vi "Hang Controller.vi"(8 "error in":errorcluster) -> ()   [LabVIEW 2019]
doc: "This VI executes continuously carrying out the current operation and responding to updates or new operations. It will often contain the timing or control code that is difficult to place directly in TeleOp. This VI generally opens all sensors and motors and isolates the rest of the robot code from knowing how the operations are carried out."
uses:
  <vilib>/Rock Robotics/WPI/Framework/Completion Status.ctl
  Hang Setpoints.ctl
  Hang Operations.ctl
  <vilib>/Rock Robotics/SystemInterfaces/DIO/FPGA_DIOPWMChannel.ctl
  <vilib>/Rock Robotics/WPI/ThirdParty/Phoenix-LabVIEW/Motor Controller/Controls/CTRE_Phoenix_MotorControl_NeutralMode.ctl
  <vilib>/Rock Robotics/WPI/ThirdParty/Phoenix-LabVIEW/Motor Controller/Controls/CTRE_Phoenix_MotorControl_TalonFXMotorControllerConfigurables.ctl
  <vilib>/Rock Robotics/WPI/ThirdParty/Phoenix-LabVIEW/Motor Controller/Controls/CTRE_Phoenix_MotorControl_BaseConfigurables.ctl
  <vilib>/Rock Robotics/WPI/ThirdParty/Phoenix-LabVIEW/Motor Controller/Controls/CTRE_Phoenix_MotorControl_VelocityMeasurementPeriod.ctl
  <vilib>/Rock Robotics/WPI/ThirdParty/Phoenix-LabVIEW/Motor Controller/Controls/CTRE_Phoenix_MotorControl_SlotStructure.ctl
  <vilib>/Rock Robotics/WPI/ThirdParty/Phoenix-LabVIEW/Motor Controller/Controls/CTRE_Phoenix_MotorControl_FilterStruct.ctl
  <vilib>/Rock Robotics/WPI/ThirdParty/Phoenix-LabVIEW/Motor Controller/Controls/CTRE_Phoenix_MotorControl_RemoteSourceType.ctl
  <vilib>/Rock Robotics/WPI/ThirdParty/Phoenix-LabVIEW/Controls/CTRE_Phoenix_CustomParamConfiguration.ctl
  <vilib>/Rock Robotics/WPI/ThirdParty/Phoenix-LabVIEW/Motor Controller/Controls/CTRE_Phoenix_MotorControl_FeedbackDevice_TalonFX.ctl
  <vilib>/Rock Robotics/WPI/ThirdParty/Phoenix-LabVIEW/Motor Controller/Controls/CTRE_Phoenix_MotorControl_LimitSwitchNormal.ctl
  <vilib>/Rock Robotics/WPI/ThirdParty/Phoenix-LabVIEW/Motor Controller/Controls/CTRE_Phoenix_MotorControl_LimitSwitchSource_Local.ctl
  <vilib>/Rock Robotics/WPI/ThirdParty/Phoenix-LabVIEW/Motor Controller/Controls/CTRE_Phoenix_MotorControl_SupplyCurrentLimitConfiguration.ctl
  <vilib>/Rock Robotics/WPI/ThirdParty/Phoenix-LabVIEW/Motor Controller/Controls/CTRE_Phoenix_MotorControl_StatorCurrentLimitConfiguration.ctl
  <vilib>/Rock Robotics/WPI/ThirdParty/Phoenix-LabVIEW/Motor Controller/Controls/CTRE_Phoenix_MotorControl_MotorCommutation_TalonFX.ctl
  <vilib>/Rock Robotics/WPI/ThirdParty/Phoenix-LabVIEW/CANCoder/Controls/CTRE_Phoenix_CANcoder_AbsoluteSensorRange.ctl
  <vilib>/Rock Robotics/WPI/ThirdParty/Phoenix-LabVIEW/CANCoder/Controls/CTRE_Phoenix_CANcoder_SensorInitializationStrategy.ctl
  <vilib>/Rock Robotics/WPI/ThirdParty/Phoenix-LabVIEW/Motor Controller/Controls/CTRE_Phoenix_MotorControl_ControlMode.ctl
  <vilib>/Rock Robotics/WPI/ThirdParty/Phoenix-LabVIEW/Motor Controller/Get/CTRE_Phoenix_MotorController_GetSelectedSensorData.vi
  <vilib>/Rock Robotics/WPI/ThirdParty/Phoenix-LabVIEW/Motor Controller/Get/CTRE_Phoenix_MotorController_GetSupplyAndStatorCurrent_Enhanced.vi
  Framework/Robot Global Data.vi
  <vilib>/Rock Robotics/Network Tables/NT Write Boolean.vi
panel:
  in  "Interactive Values":T1
  out "Current\nCmd":string
  in  "Buttons":cluster{"Execute Cmd":bool, "Abort Cmd":bool}
  out "Command Timing":cluster{"Start Time (ms)":u32, "Iterations":i32}
  out "Status":T3
  # "Tip: It may be helpful to observe inputs and sensor values.\nYou may also want to display tuning or debugging controls."
  # "Up"
  # "Down"
  # "Interactive Command: You may fill in the settings for a command\nand schedule it with the Execute button. You can observe and abort\nany command while fine tuning the code for the controller."
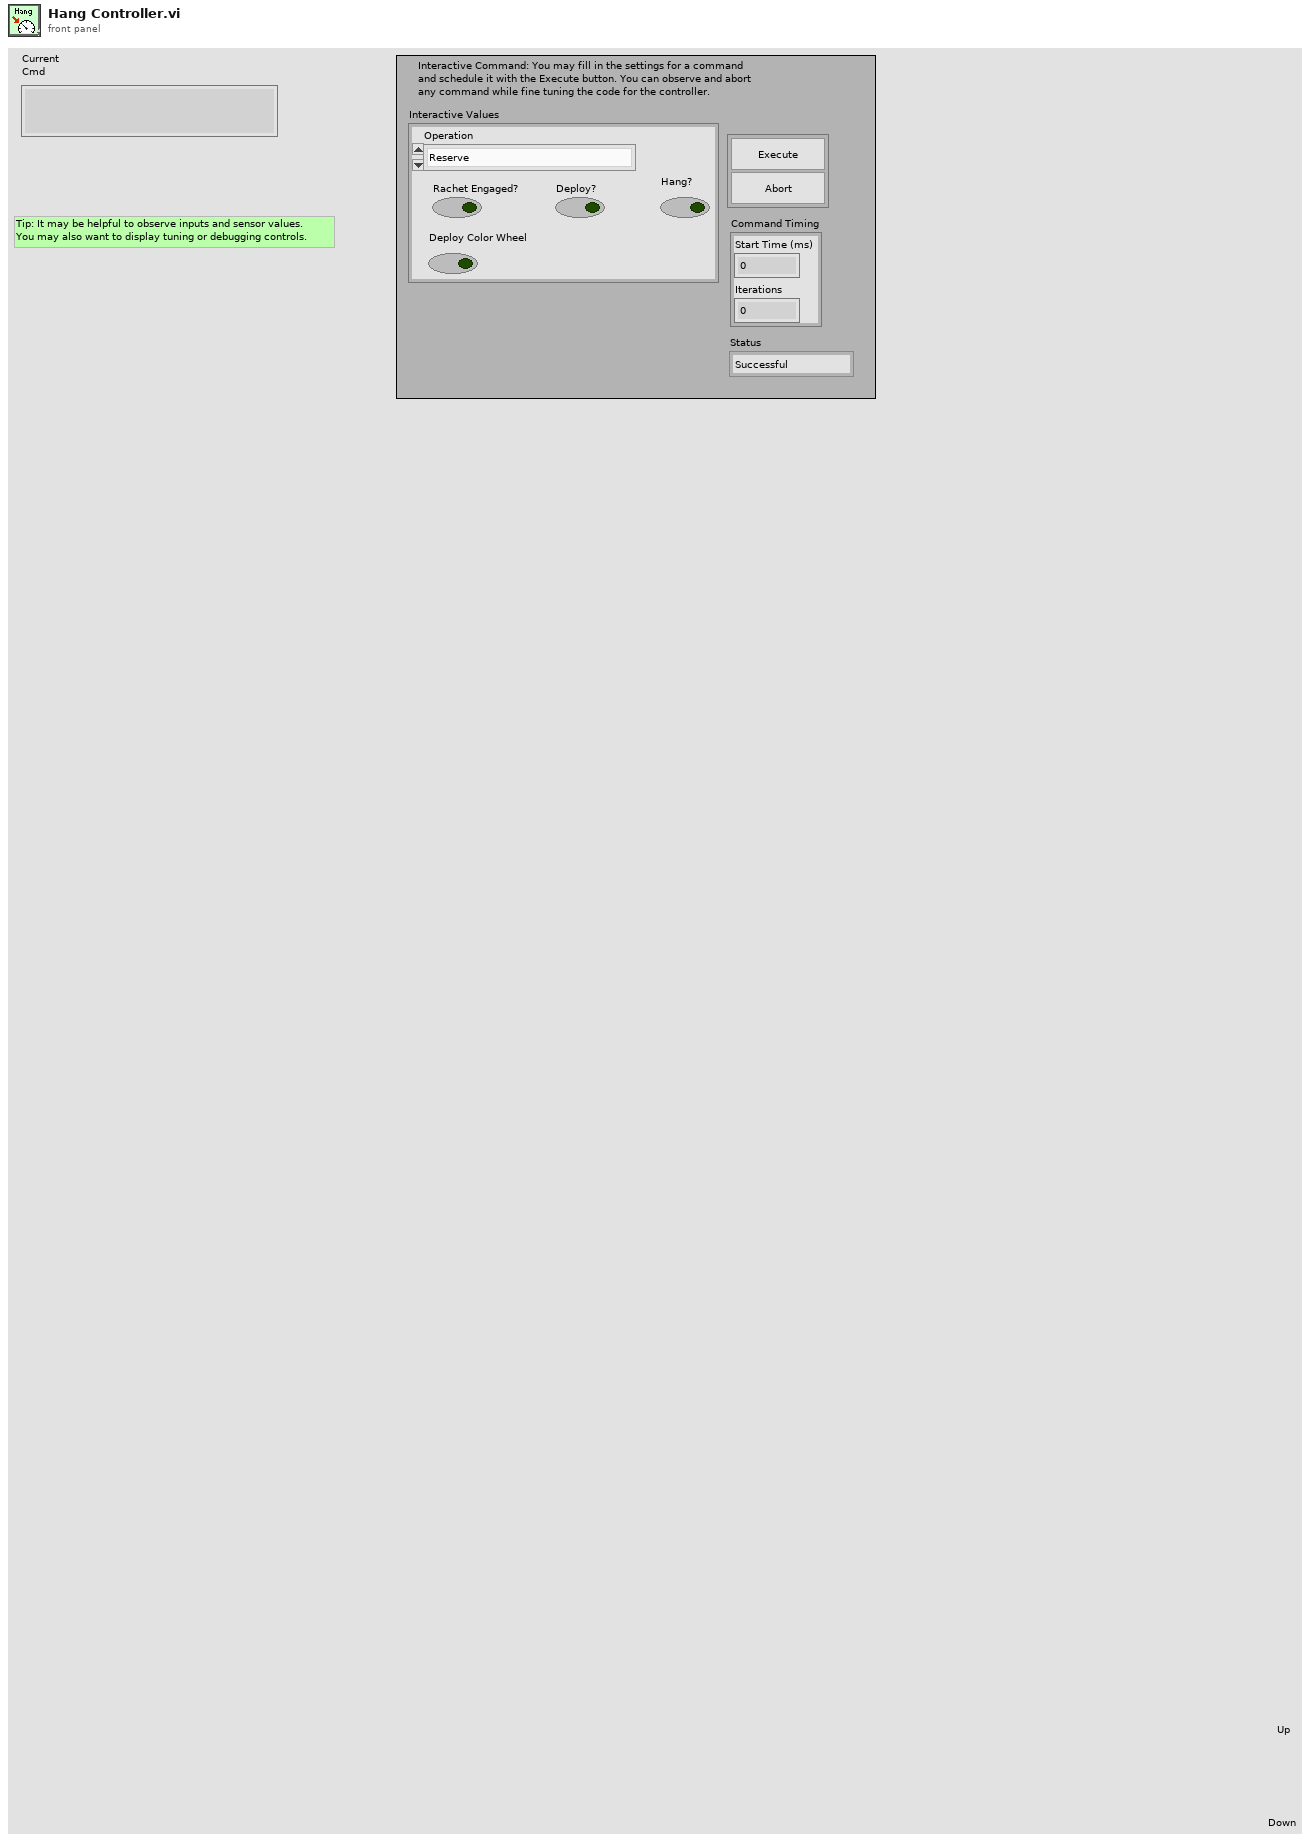
[diagram p1: front panel]
types:
  T1 = typedef "Hang Setpoints.ctl" = cluster{"Operation":T2, "Rachet Engaged?":bool, "Deploy?":bool, "Hang?":bool, "Deploy Color Wheel":bool}
  T2 = typedef "Hang Operations.ctl" = enum16{"Reserve", "Read Current", "Immediate", "Latch", "Un-Latch", "Color Wheel"}
  T3 = typedef "Completion Status.ctl" = enum16{"Successful", "Aborted", "Incomplete"}
  T4 = typedef "CTRE_Phoenix_MotorControl_TalonFXMotorControllerConfigurables.ctl" = cluster{"Base Configurables":T5, "primaryPID":cluster{"selectedFeedbackCoefficient":dbl, "selectedFeedbackSensor":T11}, "auxiliaryPID":cluster{"selectedFeedbackCoefficient":dbl, "selectedFeedbackSensor":T11}, "forwardLimitSwitchNormal":T12, "reverseLimitSwitchNormal":T12, "forwardLimitSwitchDeviceID":i32, "reverseLimitSwitchDeviceID":i32, "forwardLimitSwitchSource":T13, "reverseLimitSwitchSource":T13, "sum0Term":T11, "sum1Term":T11, "diff0Term":T11, "diff1Term":T11, "Supply Current Limit Configuration":T14, "Stator Current Limit Configuration":T15, "Motor Commutation":T16, "Absolute Sensor Range":T17, "Integrated Sensor Offset (Degrees)":dbl, "Sensor Initialization Strategy":T18}
  T5 = typedef "CTRE_Phoenix_MotorControl_BaseConfigurables.ctl" = cluster{"openLoopRamp":dbl, "closedLoopRamp":dbl, "peakOutputForward":dbl, "peakOutputReverse":dbl, "nominalOutputForward":dbl, "nominalOutputReverse":dbl, "neutralDeadband":dbl, "voltageCompSaturation":dbl, "voltageMeasurementFilter":i32, "velocityMeasurementPeriod":T6, "velocityMeasurementWindow":i32, "forwardSoftLimitThreshold":i32, "reverseSoftLimitThreshold":i32, "forwardSoftLimitEnable":bool, "reverseSoftLimitEnable":bool, "slot0":T7, "slot1":T7, "slot2":T7, "slot3":T7, "auxPIDPolarity":bool, "remoteFilter0":T8, "remoteFilter1":T8, "motionCruiseVelocity":i32, "motionAcceleration":i32, "motionProfileTrajectoryPeriod":i32, "feedbackNotContinuous":bool, "remoteSensorClosedLoopDisableNeutralOnLOS":bool, "clearPositionOnLimitF":bool, "clearPositionOnLimitR":bool, "clearPositionOnQuadIdx":bool, "limitSwitchDisableNeutralOnLOS":bool, "softLimitDisableNeutralOnLOS":bool, "pulseWidthPeriod_EdgesPerRot":i32, "pulseWidthPeriod_FilterWindowSz":i32, "customParam":T10, "trajectoryInterpolationEnable":bool}
  T6 = typedef "CTRE_Phoenix_MotorControl_VelocityMeasurementPeriod.ctl" = u16
  T7 = typedef "CTRE_Phoenix_MotorControl_SlotStructure.ctl" = cluster{"P":dbl, "I":dbl, "D":dbl, "F":dbl, "integralZone":dbl, "allowableClosedLoopError":i32, "maxIntegralAccumulator":dbl, "closedLoopPeakOutput":dbl, "closedLoopPeriod":i32}
  T8 = typedef "CTRE_Phoenix_MotorControl_FilterStruct.ctl" = cluster{"remoteSensorDeviceID":u8, "remoteSensorSource":T9}
  T9 = typedef "CTRE_Phoenix_MotorControl_RemoteSourceType.ctl" = enum16{"Off", "Talon SRX Selected Sensor", "Pigeon IMU Yaw", "Pigeon IMU Pitch", "Pigeon IMU Roll", "CANifier Quadrature", "CANifier PWM Input 0", "CANifier PWM Input 1", "CANifier PWM Input 2", "CANifier PWM Input 3", "Gadgeteer Pigeon Yaw", "Gadgeteer Pigeon Pitch", "Gadgeteer Pigeon Roll"}
  T10 = typedef "CTRE_Phoenix_CustomParamConfiguration.ctl" = cluster{"customParam0":i32, "customParam1":i32}
  T11 = typedef "CTRE_Phoenix_MotorControl_FeedbackDevice_TalonFX.ctl" = i8
  T12 = typedef "CTRE_Phoenix_MotorControl_LimitSwitchNormal.ctl" = enum16{"Normally Open", "Normally Closed", "Disabled"}
  T13 = typedef "CTRE_Phoenix_MotorControl_LimitSwitchSource_Local.ctl" = enum16{"Feedback Connector", "Remote Talon SRX", "Remote CANifier", "Deactivated"}
  T14 = typedef "CTRE_Phoenix_MotorControl_SupplyCurrentLimitConfiguration.ctl" = cluster{"Enable?":bool, "Current Limit":dbl, "Threshold Current":dbl, "Threshold Time":dbl}
  T15 = typedef "CTRE_Phoenix_MotorControl_StatorCurrentLimitConfiguration.ctl" = cluster{"Enable?":bool, "Current Limit":dbl, "Threshold Current":dbl, "Threshold Time":dbl}
  T16 = typedef "CTRE_Phoenix_MotorControl_MotorCommutation_TalonFX.ctl" = enum16{"Trapezoidal"}
  T17 = typedef "CTRE_Phoenix_CANcoder_AbsoluteSensorRange.ctl" = enum16{"Unsigned [0 to 360)", "Signed [-180 to +180)"}
  T18 = typedef "CTRE_Phoenix_CANcoder_SensorInitializationStrategy.ctl" = enum16{"Boot To Zero", "Boot To Absolute Position"}
  T19 = typedef "CTRE_Phoenix_MotorControl_NeutralMode.ctl" = enum8{"EEPROMSetting", "Override to Coast", "Override to Brake"}
  T20 = typedef "FPGA_DIOPWMChannel.ctl" = enum8{"PWM 0", "PWM 1", "PWM 2", "PWM 3", "PWM 4", "PWM 5", "PWM 6", "PWM 7", "PWM 8", "PWM 9", "PWM MXP 0", "PWM MXP 1", "PWM MXP 2", "PWM MXP 3", "PWM MXP 4", "PWM MXP 5", "PWM MXP 6", "PWM MXP 7", "PWM MXP 8", "PWM MXP 9", "Invalid"}
  T21 = typedef "WPI_MotorControlDeviceRef.ctl" = cluster{"DeviceStatus":errorcluster, "Type":T22, "PWM":cluster{"PWM Channel":T20, "DeadBand":T23}, "CAN":cluster{"Device Number":u8, "SetOutput VI Ref":variant, "GetOutput VI Ref":variant, "Enable VI Ref":variant, "Disable VI Ref":variant, "Data":variant}, "Invert":bool, "DIO PWM":cluster{"PWM \"Enable\" Channel":T20, "DIOChannel":T24, "PWM Rate":dbl}}
  T22 = typedef "WPI_MotorControlType.ctl" = enum16{"PWM", "CAN", "DIO PWM"}
  T23 = typedef "WPI_PWMDeadband.ctl" = cluster{"Name":string, "maxPositivePwm":i32, "minPositivePwm":i32, "centerPwm":i32, "maxNegativePwm":i32, "minNegativePwm":i32, "angularRange":u16}
  T24 = typedef "FPGA_DIOChannel.ctl" = enum8{"DIO 0", "DIO 1", "DIO 2", "DIO 3", "DIO 4", "DIO 5", "DIO 6", "DIO 7", "DIO 8", "DIO 9", "DIO MXP 0", "DIO MXP 1", "DIO MXP 2", "DIO MXP 3", "DIO MXP 4", "DIO MXP 5", "DIO MXP 6", "DIO MXP 7", "DIO MXP 8", "DIO MXP 9", "DIO MXP 10", "DIO MXP 11", "DIO MXP 12", "DIO MXP 13", "DIO MXP 14", "DIO MXP 15", "SPI Port CS1", "SPI Port CS2", "SPI Port CS3", "SPI Port MISO", "SPI Port MOSI", "Invalid"}
  T25 = typedef "WPI_ServoDeviceRef.ctl" = cluster{"DeviceStatus":errorcluster, "PWM Channel":T20, "DeadBand":T23}
  T26 = typedef "Command Status Info.ctl" = cluster{"Name":string, "Status":T3, "notifier out":T27}
  T27 = typedef "Completion Notifier.ctl" = refnum<notifier>
  T28 = cluster{"Current Command":T1, "Command Timing":cluster{"Start Time (ms)":u32, "Iterations":i32}, "Command Arguments":cluster{"Command Info":T26, "Description":string, "Default Command":T1, "queue out":refnum<queue>, "Subsystem Name":string}}
  T29 = enum16{"DemandType_Neutral", "DemandType_AuxPID", "DemandType_ArbitraryFeedForward"}
  T30 = typedef "CTRE_Phoenix_MotorControl_ControlMode.ctl" = u16
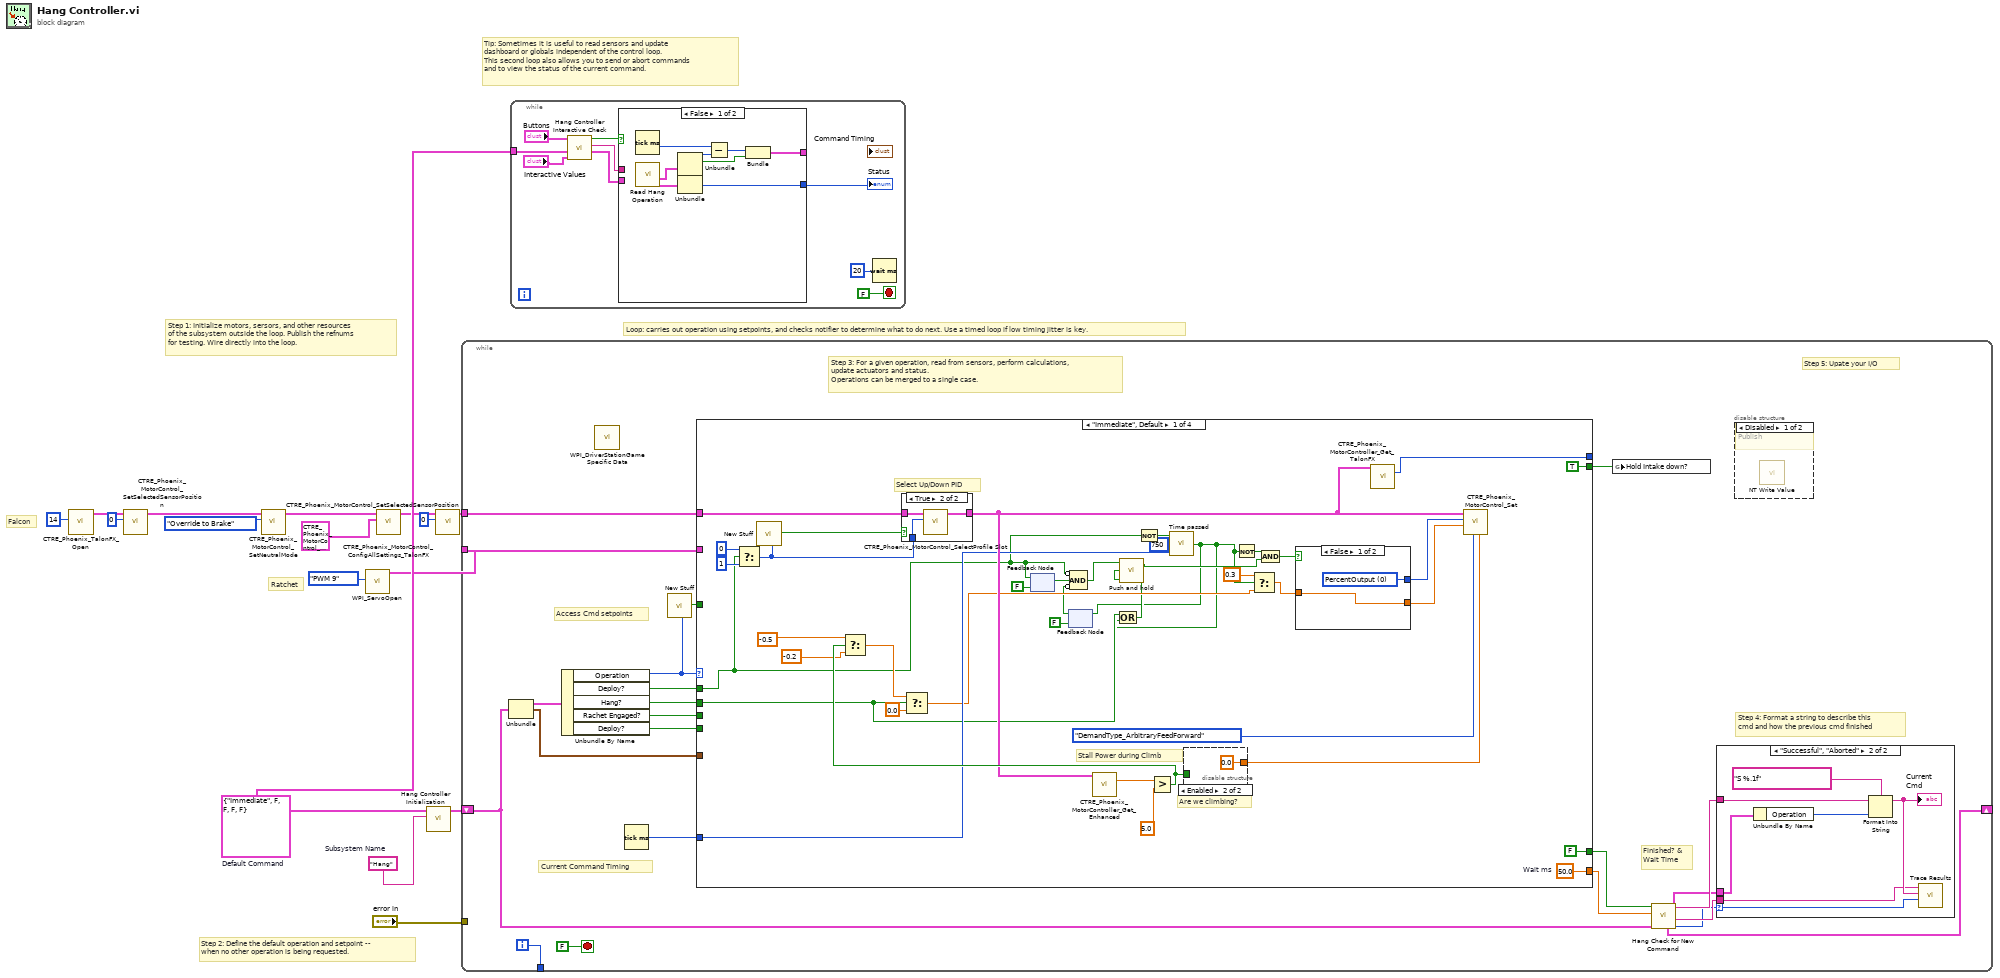
[diagram p0: block diagram]
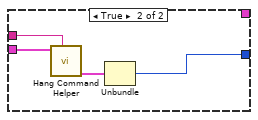
[diagram p2: hidden frame]
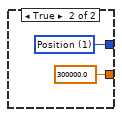
[diagram p3: hidden frame]
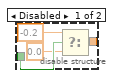
[diagram p4: hidden frame]
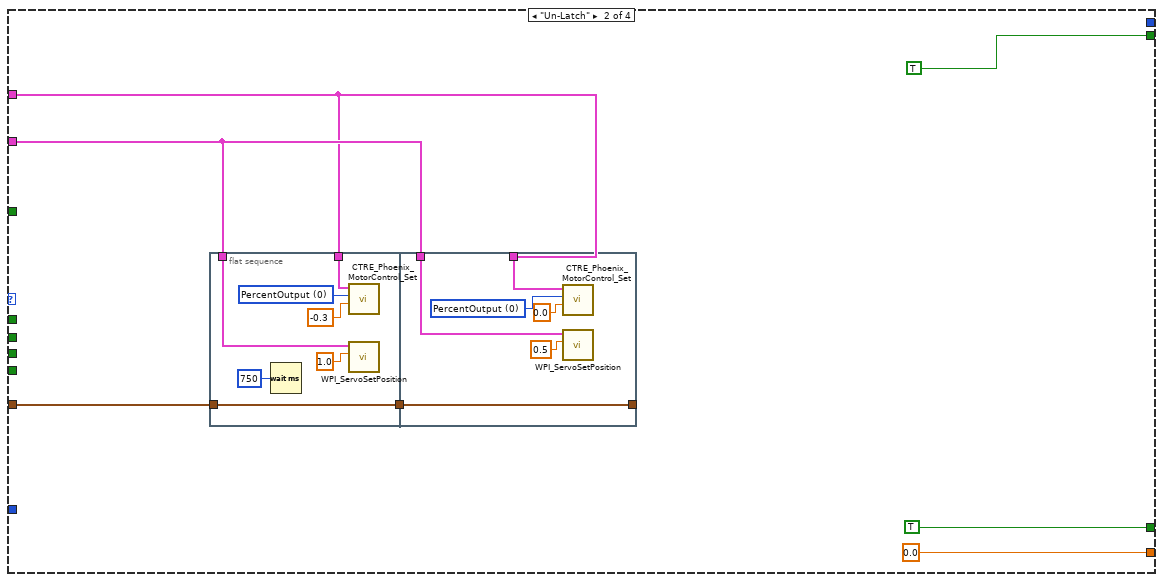
[diagram p6: hidden frame]
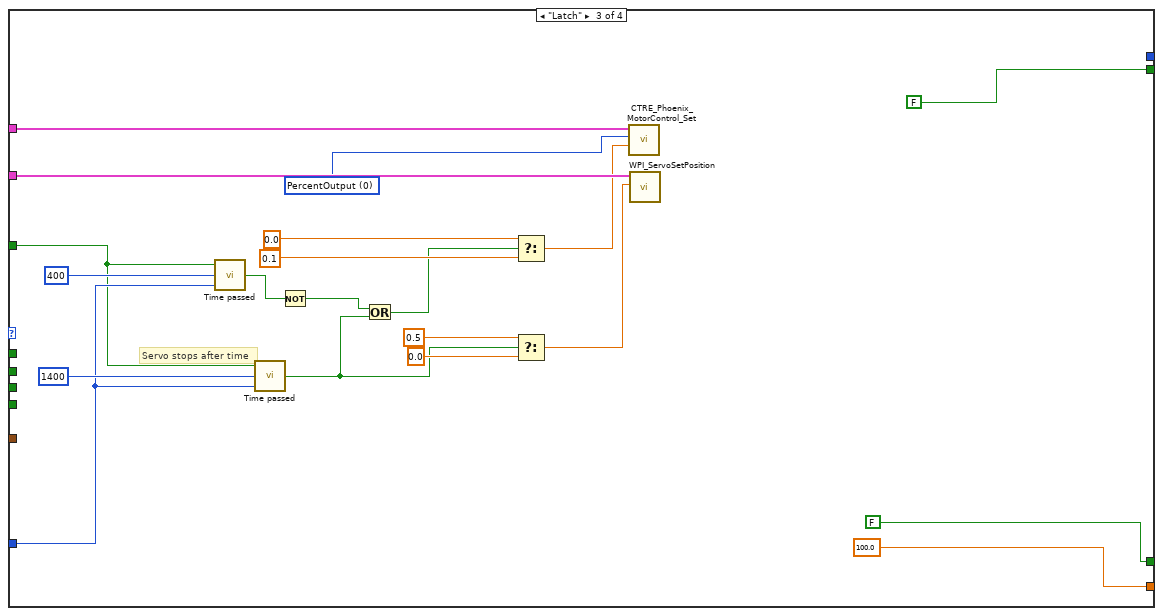
[diagram p7: hidden frame]
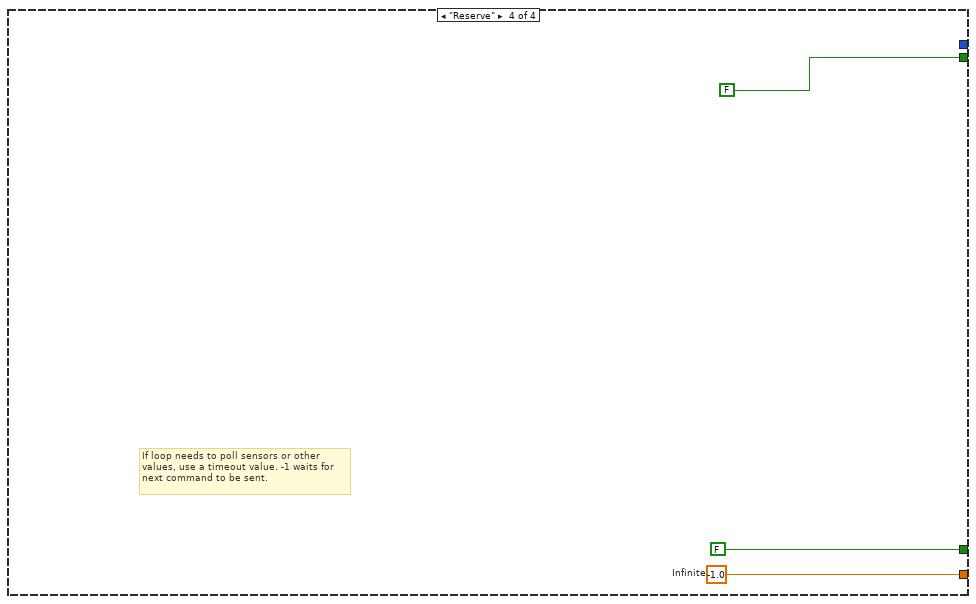
[diagram p8: hidden frame]
diagram:
  w13 = T1 {"Operation"=enum."Immediate", "Rachet Engaged?"=FALSE, "Deploy?"=FALSE, "Hang?"=FALSE, "Deploy Color Wheel"=FALSE}  # Default Command
  w14 = "Hang"  # Subsystem Name
  # "Falcon"
  # "Ratchet"
  # "Tip: Sometimes it is useful to read sensors and update\ndashboard or globals independent of the control loop.\nThis second loop also allows you to send or abort commands\nand to view the status of the current command."
  # "Step 2: Define the default operation and setpoint --\nwhen no other operation is being requested."
  # "Step 1: Initialize motors, sersors, and other resources\nof the subsystem outside the loop. Publish the refnums\nfor testing. Wire directly into the loop."
  # "Loop: carries out operation using setpoints, and checks notifier to determine what to do next. Use a timed loop if low timing jitter is key."
  n1 = call <vilib>:"CTRE_Phoenix_TalonFX_Open.vi"("Device Number"=u8 14) -> ("CAN Talon SRX Ref"=w9:T21)  [unwired: 9 in, 1 out]
  n2 = call <vilib>:"CTRE_Phoenix_MotorControl_SetSelectedSensorPosition.vi"("New Sensor Position"=0, "PhoenixMotorControlDevRef"=w9) -> ("PhoenixMotorControlDevRef"=w6:T21)  [unwired: 8 in, 1 out]
  n3 = call <vilib>:"CTRE_Phoenix_MotorControl_SetNeutralMode.vi"("Motor Control Neutral Mode"=CTRE_Phoenix_MotorControl_NeutralMode."Override to Brake", "PhoenixMotorControlDevRef"=w6) -> ("PhoenixMotorControlDevRef"=w3:T21)  [unwired: 8 in, 1 out]
  n4 = call <vilib>:"WPI_ServoOpen.vi"("PWM Channel"=FPGA_DIOPWMChannel."PWM 9") -> ("ServoDeviceRef"=w11:T25)  [unwired: 9 in, 1 out]
  n5 = call <vilib>:"CTRE_Phoenix_MotorControl_ConfigAllSettings_TalonFX.vi"("Talon FX Configurables"=T4 {"Base Configurables"={"openLoopRamp"=0.0, "closedLoopRamp"=0.0, "peakOutputForward"=1.0, "peakOutputReverse"=-1.0, "nominalOutputForward"=0.0, "nominalOutputReverse"=0.0, "neutralDeadband"=0.04, "voltageCompSaturation"=0.0, "voltageMeasurementFilter"=32, "velocityMeasurementPeriod"=100, "velocityMeasurementWindow"=64, "forwardSoftLimitThreshold"=0, "reverseSoftLimitThreshold"=0, "forwardSoftLimitEnable"=FALSE, "reverseSoftLimitEnable"=FALSE, "slot0"={"P"=0.04, "I"=5e-05, "D"=0.0, "F"=0.0, "integralZone"=20000.0, "allowableClosedLoopError"=0, "maxIntegralAccumulator"=0.0, "closedLoopPeakOutput"=0.7, "closedLoopPeriod"=1}, "slot1"={"P"=0.05, "I"=5e-05, "D"=0.0, "F"=0.0, "integralZone"=20000.0, "allowableClosedLoopError"=0, "maxIntegralAccumulator"=0.0, "closedLoopPeakOutput"=1.0, "closedLoopPeriod"=1}, "slot2"={"P"=0.0, "I"=0.0, "D"=0.0, "F"=0.0, "integralZone"=0.0, "allowableClosedLoopError"=0, "maxIntegralAccumulator"=0.0, "closedLoopPeakOutput"=1.0, "closedLoopPeriod"=1}, "slot3"={"P"=0.0, "I"=0.0, "D"=0.0, "F"=0.0, "integralZone"=0.0, "allowableClosedLoopError"=0, "maxIntegralAccumulator"=0.0, "closedLoopPeakOutput"=1.0, "closedLoopPeriod"=1}, "auxPIDPolarity"=FALSE, "remoteFilter0"={"remoteSensorDeviceID"=0, "remoteSensorSource"=enum."Off"}, "remoteFilter1"={"remoteSensorDeviceID"=0, "remoteSensorSource"=enum."Off"}, "motionCruiseVelocity"=0, "motionAcceleration"=0, "motionProfileTrajectoryPeriod"=0, "feedbackNotContinuous"=FALSE, "remoteSensorClosedLoopDisableNeutralOnLOS"=FALSE, "clearPositionOnLimitF"=FALSE, "clearPositionOnLimitR"=FALSE, "clearPositionOnQuadIdx"=FALSE, "limitSwitchDisableNeutralOnLOS"=FALSE, "softLimitDisableNeutralOnLOS"=FALSE, "pulseWidthPeriod_EdgesPerRot"=1, "pulseWidthPeriod_FilterWindowSz"=1, "customParam"={"customParam0"=0, "customParam1"=0}, "trajectoryInterpolationEnable"=TRUE}, "primaryPID"={"selectedFeedbackCoefficient"=1.0, "selectedFeedbackSensor"=1}, "auxiliaryPID"={"selectedFeedbackCoefficient"=1.0, "selectedFeedbackSensor"=1}, "forwardLimitSwitchNormal"=enum."Normally Open", "reverseLimitSwitchNormal"=enum."Normally Open", "forwardLimitSwitchDeviceID"=0, "reverseLimitSwitchDeviceID"=0, "forwardLimitSwitchSource"=enum."Feedback Connector", "reverseLimitSwitchSource"=enum."Feedback Connector", "sum0Term"=1, "sum1Term"=1, "diff0Term"=1, "diff1Term"=1, "Supply Current Limit Configuration"={"Enable?"=FALSE, "Current Limit"=0.0, "Threshold Current"=0.0, "Threshold Time"=0.0}, "Stator Current Limit Configuration"={"Enable?"=FALSE, "Current Limit"=0.0, "Threshold Current"=0.0, "Threshold Time"=0.0}, "Motor Commutation"=enum."Trapezoidal", "Absolute Sensor Range"=enum."Unsigned [0 to 360)", "Integrated Sensor Offset (Degrees)"=0.0, "Sensor Initialization Strategy"=enum."Boot To Zero"}, "PhoenixMotorControlDevRef"=w3) -> ("PhoenixMotorControlDevRef"=w2:T21)  [unwired: 8 in, 1 out]
  n6 = call "Hang Controller Initialization.vi"("Subsystem Name"=w14, "Default Command"=w13) -> ("Current Command"=w15:T28)  [unwired: 9 in]
  n7 = call <vilib>:"CTRE_Phoenix_MotorControl_SetSelectedSensorPosition.vi"("New Sensor Position"=0, "PhoenixMotorControlDevRef"=w2) -> ("PhoenixMotorControlDevRef"=w5:T21)  [unwired: 8 in, 1 out]
  n8 = while {
    shift-right: [w31] -> _
    shift-left: w15 -> [w24]
    tunnel: [w37] -> _
    tunnel: "error in" -> [_]
    tunnel: w11 -> [w22]
    tunnel: w5 -> [w17]
    i -> [w37]
    stop <- FALSE stop-if-true
    # "Step 5: Upate your I/O"
    # "Step 4: Format a string to describe this\ncmd and how the previous cmd finished"
    # "Current Command Timing"
    # "Access Cmd setpoints"
    # "Finished? &\nWait Time"
    # "Step 3: For a given operation, read from sensors, perform calculations,\nupdate actuators and status.\nOperations can be merged to a single case."
    n9 = Unbundle(w24) -> ("Current Command"=w36:T1, "Command Timing"=w33:cluster{"Start Time (ms)":u32, "Iterations":i32})  [unwired: 1 out]
    n10 = Unbundle By Name(w36) -> ("Operation"=w20:T2, "Deploy?"=w35:bool, "Hang?"=w32:bool, "Rachet Engaged?"=w23:bool, "Deploy?"=w21:bool)
    n11 = call <vilib>:"WPI_DriverStationGame Specific Data.vi"() -> ()  [unwired: 11 in, 1 out]
    n12 = Tick Count (ms)() -> (millisecond timer value=w34:u32)
    n13 = call "New Stuff.vi"("Variant 9"=w20) -> ("x != y?"=w19:bool)  [unwired: 26 in]
    n14 = case shown="\"Immediate\", Default" w20 {
      tunnel: [w77 0.0 ("Infinite") 100.0 ("Infinite") w133] -> w29
      tunnel: [FALSE ("ignore previous (F)") TRUE ("ignore previous (F)") FALSE ("ignore previous (F)") FALSE ("ignore previous (F)")] -> w30
      tunnel: w33 -> [_ w96 _ _]
      tunnel: w35 -> [w43 _ _ _]
      tunnel: w34 -> [w55 _ w118 _]
      tunnel: w32 -> [w47 _ _ _]
      tunnel: w23 -> [_ _ _ _]
      tunnel: w22 -> [_ w97 w128 _]
      tunnel: w21 -> [_ _ _ _]
      tunnel: w19 -> [_ _ w116 _]
      tunnel: w17 -> [w64 w92 w126 _]
      tunnel: [TRUE ("Hold Intake down?") TRUE ("Hold Intake down?") FALSE ("Hold Intake down?") FALSE ("Hold Intake down?")] -> w18
      tunnel: [w58 _ _ _] -> _
      frame "Immediate", Default {
        w77 = 50.0  # Wait ms
        # "Select Up/Down PID"
        # "Stall Power during Climb"
        # "Are we climbing?"
        n15 = Select(t=0 ("slotIdx"), s=w43, f=1 ("slotIdx")) -> (s? t:f=w66:i32)
        n16 = call "New Stuff.vi"("Variant 9"=w66) -> ("x != y?"=w65:bool)  [unwired: 26 in]
        n17 = case shown="True" w65 {
          tunnel: [w87 w90] -> w59
          tunnel: w64 -> [w87 w89]
          tunnel: w66 -> [_ w88]
          frame False {
          }
          frame True {
            n18 = call <vilib>:"CTRE_Phoenix_MotorControl_SelectProfile Slot.vi"("slotIdx"=w88, "PhoenixMotorControlDevRef"=w89) -> ("PhoenixMotorControlDevRef"=w90:T21)  [unwired: 8 in, 1 out]
          }
        }
        n19 = feedback-in #1(w43) -> ()
        n20 = feedback #1(FALSE ("Deploy?")) -> (w44:bool)
        n21 = feedback #2(FALSE ("Boolean out")) -> (w41:bool)
        n22 = Compound Arithmetic op=AND(invert w43, w44, invert w41) -> (w42:bool)
        n23 = call-poly <vilib>:"CTRE_Phoenix_MotorController_Get_Enhanced.vi"("PhoenixMotorControlDevRef"=w59) -> ("Supply Current"=w73:dbl)  [unwired: 11 in, 3 out]
        n24 = Not(x=w43) -> (.not. x?=w56:bool)
        n25 = Greater?(x=w73, y=5.0 ("Current")) -> (0:w62:bool)
        n26 = Select(t=-0.5 ("Main Down 3"), s=w62, f=-0.2 ("Main Down 2")) -> (s? t:f=w76:dbl)
        n27 = Select(t=w76, s=w47, f=0.0) -> (s? t:f=w49:dbl)
        n28 = call "Time passed.vi"("ms timer value"=w55, "Wait time"=u32 750, "Reset"=w56) -> ("Boolean out"=w40:bool)
        n29 = feedback-in #2(w40) -> ()
        n30 = Or(x=w47, y=w40) -> (x .or. y?=w46:bool)
        n31 = call "Push and hold.vi"("Reset"=w46, "Input"=w42) -> ("Output"=w53:bool)  [unwired: 2 in]
        n32 = disable-structure shown="Enabled" {
          disable-tunnel: w62 -> [w85 _]
          disable-tunnel: [w84 0.0 ("Demand1")] -> w69
          frame Disabled {
            n33 = Select(t=-0.2 ("AFF"), s=w85, f=0.0 ("AFF")) -> (s? t:f=w84:dbl)
          }
          frame Enabled {
          }
        }
        n34 = Not(x=w40) -> (.not. x?=w52:bool)
        n35 = Select(t=0.3, s=w40, f=w49) -> (s? t:f=w48:dbl)
        n36 = And(x=w52, y=w53) -> (x .and. y?=w51:bool)
        n37 = case shown="False" w51 {
          tunnel: [w79 w81] -> w68
          tunnel: w48 -> [w78 _]
          tunnel: [w78 300000.0 ("f")] -> w57
          frame False {
            w79 = T30 0 items=["PercentOutput"=0, "Position"=1, "Velocity"=2, "Current"=3, "Follower"=5, "MotionProfile"=6, "MotionMagic"=7, "MotionProfileArc"=10, "Disabled"=15] ("Control Mode")
          }
          frame True {
            w81 = T30 1 items=["PercentOutput"=0, "Position"=1, "Velocity"=2, "Current"=3, "Follower"=5, "MotionProfile"=6, "MotionMagic"=7, "MotionProfileArc"=10, "Disabled"=15] ("Control Mode")
          }
        }
        n38 = call-poly <vilib>:"CTRE_Phoenix_MotorController_Get_TalonFX.vi"("PhoenixMotorControlDevRef"=w59) -> ("Position (Raw Sensor Units)"=w58:i32)  [unwired: 11 in, 3 out]
        n39 = call <vilib>:"CTRE_Phoenix_MotorControl_Set.vi"("Demand1"=w69, "DemandType"=T29."DemandType_ArbitraryFeedForward", "Output"=w57, "Control Mode"=w68, "PhoenixMotorControlDevRef"=w59) -> ()  [unwired: 5 in, 2 out]
      }
      frame "Un-Latch" {
        n40 = flat-sequence {
          tunnel: w97 -> [w101]
          tunnel: w96 -> [w103]
          tunnel: [w103] -> w93
          tunnel: w92 -> [w100]
          tunnel: w97 -> [w108]
          tunnel: w93 -> [w110]
          tunnel: [w110] -> _
          tunnel: w92 -> [w105]
          frame #0 {
            w98 = T30 0 items=["PercentOutput"=0, "Position"=1, "Velocity"=2, "Current"=3, "Follower"=5, "MotionProfile"=6, "MotionMagic"=7, "MotionProfileArc"=10, "Disabled"=15] ("Control Mode")
            n41 = Wait (ms)(milliseconds to wait=u32 750) -> ()  [unwired: 1 out]
            n42 = call <vilib>:"CTRE_Phoenix_MotorControl_Set.vi"("Output"=-0.3 ("Un POW 1"), "Control Mode"=w98, "PhoenixMotorControlDevRef"=w100) -> ()  [unwired: 7 in, 2 out]
            n43 = call <vilib>:"WPI_ServoSetPosition.vi"("Position"=1.0, "ServoDeviceRef"=w101) -> ()  [unwired: 8 in, 2 out]
          }
          frame #1 {
            w106 = T30 0 items=["PercentOutput"=0, "Position"=1, "Velocity"=2, "Current"=3, "Follower"=5, "MotionProfile"=6, "MotionMagic"=7, "MotionProfileArc"=10, "Disabled"=15] ("Control Mode")
            n44 = call <vilib>:"CTRE_Phoenix_MotorControl_Set.vi"("Output"=0.0, "Control Mode"=w106, "PhoenixMotorControlDevRef"=w105) -> ()  [unwired: 7 in, 2 out]
            n45 = call <vilib>:"WPI_ServoSetPosition.vi"("Position"=0.5, "ServoDeviceRef"=w108) -> ()  [unwired: 8 in, 2 out]
          }
        }
      }
      frame "Latch" {
        w125 = T30 0 items=["PercentOutput"=0, "Position"=1, "Velocity"=2, "Current"=3, "Follower"=5, "MotionProfile"=6, "MotionMagic"=7, "MotionProfileArc"=10, "Disabled"=15] ("Control Mode")
        # "Servo stops after time"
        n46 = call "Time passed.vi"("ms timer value"=w118, "Wait time"=u32 400, "Reset"=w116) -> ("Boolean out"=w112:bool)
        n47 = call "Time passed.vi"("ms timer value"=w118, "Wait time"=u32 1400, "Reset"=w116) -> ("Boolean out"=w114:bool)
        n48 = Not(x=w112) -> (.not. x?=w111:bool)
        n49 = Or(x=w111, y=w114) -> (x .or. y?=w115:bool)
        n50 = Select(t=0.0, s=w115, f=0.1) -> (s? t:f=w121:dbl)
        n51 = Select(t=0.5 ("Position"), s=w114, f=0.0 ("Position")) -> (s? t:f=w122:dbl)
        n52 = call <vilib>:"CTRE_Phoenix_MotorControl_Set.vi"("Output"=w121, "Control Mode"=w125, "PhoenixMotorControlDevRef"=w126) -> ()  [unwired: 7 in, 2 out]
        n53 = call <vilib>:"WPI_ServoSetPosition.vi"("Position"=w122, "ServoDeviceRef"=w128) -> ()  [unwired: 8 in, 2 out]
      }
      frame "Reserve" {
        w133 = -1.0  # Infinite
        # "If loop needs to poll sensors or other\nvalues, use a timeout value. -1 waits for\nnext command to be sent."
      }
    }
    n54 = global write "Robot Global Data.vi" "Hold Intake down?"(w18) -> ()
    n55 = call "Hang Check for New Command.vi"("Current Command"=w24, "Wait time (ms)"=w29, "Finished?"=w30) -> ("Completion"=w25:T3, "Subsystem Name"=w26:string, "Current Command"=w27:T1, "Initial Trace String"=w28:string, "NextCommand"=w31:T28)  [unwired: 4 in]
    n56 = case shown="\"Successful\", \"Aborted\"" w25 {
      selector: w25 -> [_ w140]
      tunnel: w28 -> [_ w136]
      tunnel: w27 -> [_ w137]
      tunnel: w26 -> [_ w134]
      frame "Incomplete", Default {
        # "Continuing current command"
      }
      frame "Successful", "Aborted" {
        # "Report and setup for next command"
        n57 = Unbundle By Name(w137) -> ("Operation"=w139:T2)
        n58 = Format Into String(format string="S %.1f", initial string=w136, w139) -> (resulting string=w135:string)  [unwired: 1 in, 1 out]
        "Current\nCmd" <- w135
        n59 = call <vilib>:"Trace Results.vi"("Status of previous command"=w140, "Description"=w135, "Subsystem"=w134) -> ()  [unwired: 9 in]
      }
    }
    n60 = disable-structure shown="Disabled" {
      frame Disabled {
        # "Publish"
        n61 = call-poly <vilib>:"NT Write Value.vi"() -> ()  [unwired: 11 in, 1 out]
      }
      frame Enabled {
      }
    }
  }
  n62 = while {
    tunnel: w13 -> [w146]
    stop <- FALSE stop-if-true
    n63 = call "Hang Controller Interactive Check.vi"("Interactive Command in"="Interactive Values", "Default Command"=w146, "Buttons"="Buttons") -> ("Interactive Command out"=w143:T1, "Trace String"=w144:string, "Schedule"=w145:bool)  [unwired: 6 in]
    n64 = case shown="False" w145 {
      tunnel: [w157 w161] -> w142
      tunnel: w143 -> [_ w159]
      tunnel: [w153 _] -> _
      tunnel: w144 -> [_ w160]
      frame False {
        n65 = Tick Count (ms)() -> (millisecond timer value=w152:u32)
        n66 = call "Read Hang Operation.vi"() -> ("Command Info"=w150:T26, "SubSystem Data"=w151:T1)  [unwired: 9 in, 1 out]
        n67 = Unbundle(w151) -> ("Operation"=w156:T2, "Rachet Engaged?"=w154:bool)  [unwired: 3 out]
        n68 = Unbundle(w150) -> ("Status"=w157:T3)  [unwired: 2 out]
        n69 = Subtract(x=w152, y=w156) -> (x-y=w155:u32)
        n70 = Bundle(w155, "Rachet Engaged?"=w154) -> (w153:cluster{u32, "Rachet Engaged?":bool})  [unwired: 1 in]
      }
      frame True {
        n71 = call "Hang Command Helper.vi"("Description"=w160, "SubSystem Data"=w159) -> ("Command Info Out"=w158:T26)  [unwired: 7 in, 2 out]
        n72 = Unbundle(w158) -> ("Status"=w161:T3)  [unwired: 2 out]
      }
    }
    "Status" <- w142
    n73 = Wait (ms)(milliseconds to wait=u32 20) -> ()  [unwired: 1 out]
  }
